vi "fpga_U16counter.vi"(9 "input valid":bool=TRUE, 11 "reset":bool) -> (3 "Counter":u16)   [LabVIEW 2011, in "NI_EP_Resample_FPGA.lvlib"]
uses:
  <vilib>/rvi/FXPMathLib/basic elements/FxpAddSub/XNode/nifxpmath_AddSub.xnode
  <vilib>/addons/Electrical Power/PQ/Resampling/NI_EP_Resample_FPGA.lvlib
  <vilib>/rvi/FXPMathLib/sim/FxpSim.dll
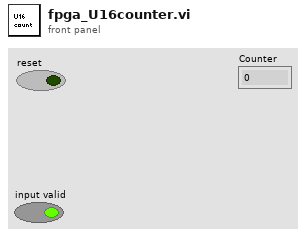
[diagram p1: front panel]
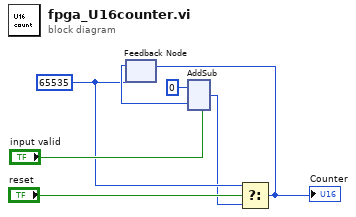
[diagram p0: block diagram]
diagram:
  w4 = u16 65535 ("s")
  n1 = feedback #1(w4) -> (w7:u16)
  n2 = xnode "AddSub"("x"=u16 0, "y"=w7, "carry-in"="input valid") -> ("s"=w1:u16)  [unwired: 1 out]
  n3 = Select(t=w4, s="reset", f=w1) -> (s? t:f=w3:u16)
  "Counter" <- w3
  n4 = feedback-in #1(w3) -> ()
